vi "F510-X.vi"(7 "Smooth Control (T)":bool=TRUE, 8 "error in (no error)":errorcluster, 10 "Deadzone Scale Cluster":cluster{"Scale":dbl, "Deadzone":dbl}={"Scale"=1.0, "Deadzone"=0.1}, 11 "refnum name":string) -> (0 "error out":errorcluster, 1 "Right Stick":cluster{"X":dbl, "Y":dbl}, 2 "Left Stick":cluster{"X":dbl, "Y":dbl}, 3 "JoystickDevRef":T2, 4 "Buttons":T1, 5 "Triggers":cluster{"Left":dbl, "Right":dbl}, 6 "D-Pad Buttons":T4)   [LabVIEW 2015]
uses:
  <vilib>/Rock Robotics/WPI/Joystick/WPI_JoystickDevRef.ctl
  <vilib>/Rock Robotics/WPI/Joystick/WPI_JoystickDeviceEnum.ctl
  <vilib>/Rock Robotics/WPI/Utilities/WPI_GetSetVariantRefNum.vi
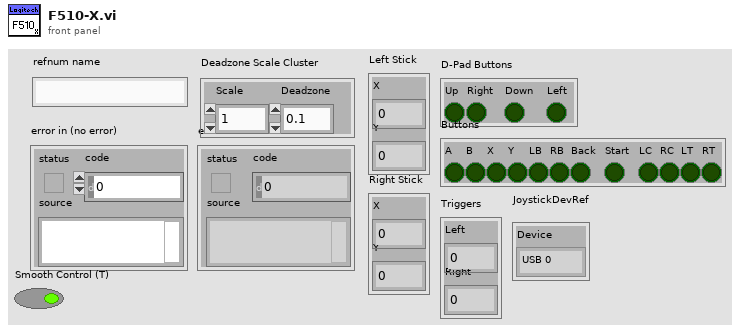
[diagram p1: front panel]
types:
  T1 = cluster{"A":bool, "B":bool, "X":bool, "Y":bool, "LB":bool, "RB":bool, "Back":bool, "Start":bool, "LC":bool, "RC":bool, "LT":bool, "RT":bool}
  T2 = typedef "WPI_JoystickDevRef.ctl" = cluster{"Device":T3}
  T3 = typedef "WPI_JoystickDeviceEnum.ctl" = enum16{"USB 0", "USB 1", "USB 2", "USB 3", "USB 4", "USB 5"}
  T4 = cluster{"Up":bool, "Right":bool, "Down":bool, "Left":bool}
  T5 = cluster{"[0]":dbl, "[1]":dbl, "[2]":dbl, "[3]":dbl, "[4]":dbl, "[5]":dbl}
  T6 = cluster{"Buttons[0]":bool, "Buttons[1]":bool, "Buttons[2]":bool, "Buttons[3]":bool, "Buttons[4]":bool, "Buttons[5]":bool, "Buttons[6]":bool, "Buttons[7]":bool, "Buttons[8]":bool, "Buttons[9]":bool}
  T7 = cluster{"Up":bool, "Down":bool, "Left":bool, "Right":bool}[]
  T8 = cluster{"Up":bool, "Down":bool, "Left":bool, "Right":bool}
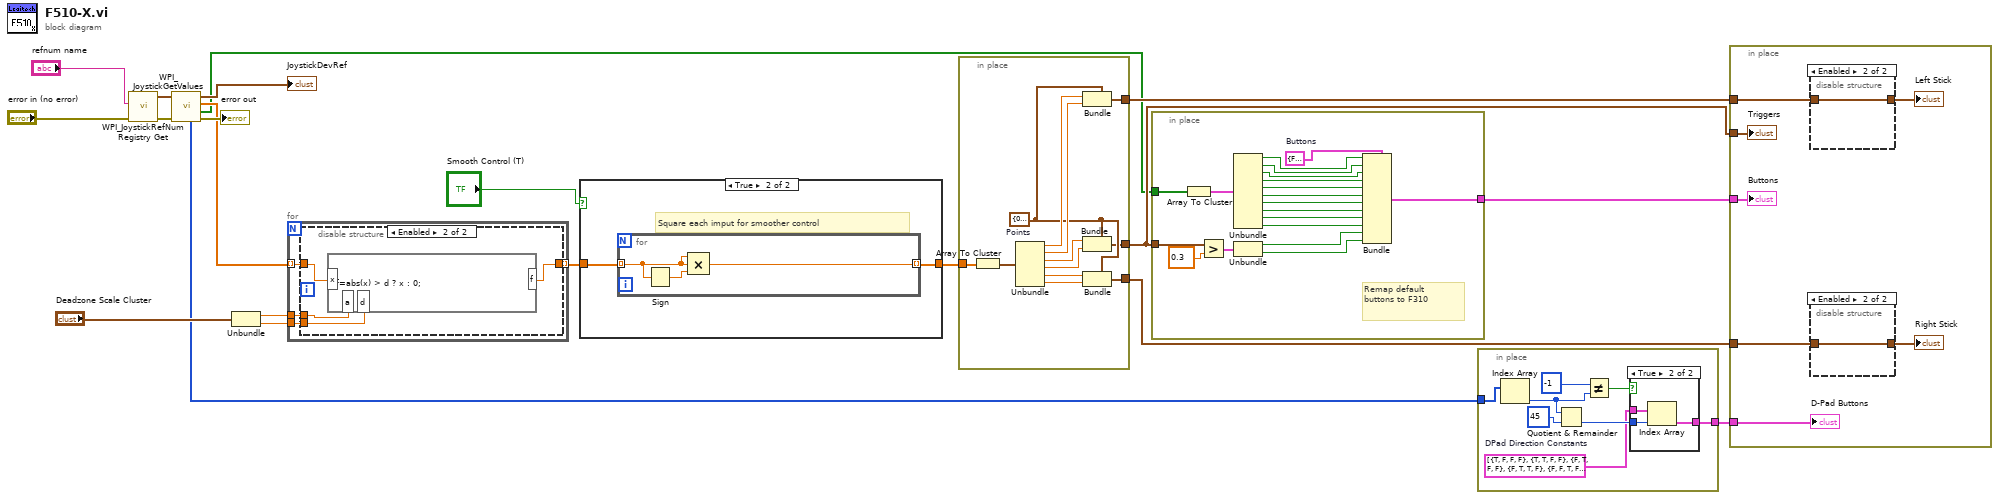
[diagram p0: block diagram]
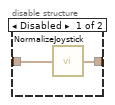
[diagram p3: hidden frame]
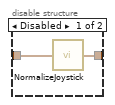
[diagram p4: hidden frame]
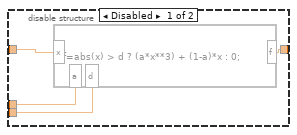
[diagram p6: hidden frame]
diagram:
  n1 = call <vilib>:"WPI_JoystickRefNum Registry Get.vi"("error in (no error)"="error in (no error)", "refnum name"="refnum name") -> ("error out"=w17:errorcluster, "JoystickDevRef"=w18:T2)  [unwired: 8 in]
  n2 = call <vilib>:"WPI_JoystickGetValues.vi"("error in (no error)"=w17, "JoystickDevRef"=w18) -> ("error out"=→"error out":errorcluster, "Buttons"=w5:bool[], "Axes"=w15:dbl[], "JoystickDevRef"=→"JoystickDevRef":T2, "POVs"=w9:i16[])  [unwired: 5 in]
  n3 = Unbundle("Deadzone Scale Cluster") -> ("Scale"=w13:dbl, "Deadzone"=w12:dbl)
  n4 = for {
    tunnel: w15 -> [w24] mode=indexing
    tunnel: w13 -> [w23]
    tunnel: w12 -> [w22]
    tunnel: [w21] -> w1 mode=indexing
    n5 = disable-structure shown="Enabled" {
      disable-tunnel: w24 -> [w28 w30]
      disable-tunnel: w23 -> [w27 w32]
      disable-tunnel: w22 -> [w26 w31]
      disable-tunnel: [w25 w29] -> w21
      frame Disabled {
        n6 = formula code="f=abs(x) > d ? (a*x**3) + (1-a)*x : 0;"("x"=w28, "d"=w26, "a"=w27) -> ("f"=w25:dbl)
      }
      frame Enabled {
        n7 = formula code="f=abs(x) > d ? x : 0;"("x"=w30, "d"=w31, "a"=w32) -> ("f"=w29:dbl)
      }
    }
  }
  n8 = case shown="True" "Smooth Control (T)" {
    tunnel: [w33 w35] -> w2
    tunnel: w1 -> [w33 w34]
    frame False {
    }
    frame True {
      # "Square each imput for smoother control"
      n9 = for {
        tunnel: [w38] -> w35 mode=indexing
        tunnel: w34 -> [w37] mode=indexing
        n10 = Sign(1:w37) -> (0:w36:dbl)
        n11 = Compound Arithmetic op=MULTIPLY(w37, w37, w36) -> (w38:dbl)
      }
    }
  }
  n12 = in-place {
    in-place-border: w2 -> [w47]
    in-place-border: [w43] -> w10
    in-place-border: [w46] -> w11
    in-place-border: [w41] -> w8
    w42 = cluster{"X":dbl, "Y":dbl} {"X"=0.0, "Y"=0.0}  # Points
    n13 = Array To Cluster(array=w47) -> (cluster=w50:T5)
    n14 = Unbundle(w50) -> ("[0]"=w48:dbl, "[1]"=w49:dbl, "[2]"=w40:dbl, "[3]"=w39:dbl, "[4]"=w45:dbl, "[5]"=w44:dbl)
    n15 = Bundle(cluster=w42, "X"=w48, "Y"=w49) -> (w46:cluster{"X":dbl, "Y":dbl})
    n16 = Bundle(cluster=w42, "X"=w40, "Y"=w39) -> (w41:cluster{"X":dbl, "Y":dbl})
    n17 = Bundle(cluster=w42, "X"=w45, "Y"=w44) -> (w43:cluster{"X":dbl, "Y":dbl})
  }
  n18 = in-place {
    in-place-border: w5 -> [w60]
    in-place-border: [w62] -> w4
    in-place-border: w8 -> [w55]
    w69 = T1 {"A"=FALSE, "B"=FALSE, "X"=FALSE, "Y"=FALSE, "LB"=FALSE, "RB"=FALSE, "Back"=FALSE, "Start"=FALSE, "LC"=FALSE, "RC"=FALSE, "LT"=FALSE, "RT"=FALSE}  # Buttons
    # "Remap default\nbuttons to F310"
    n19 = Array To Cluster(array=w60) -> (cluster=w61:T6)
    n20 = Greater?(x=w55, y=0.3) -> (0:w53:cluster{"X":bool, "Y":bool})
    n21 = Unbundle(w61) -> ("Buttons[0]"=w68:bool, "Buttons[1]"=w67:bool, "Buttons[2]"=w66:bool, "Buttons[3]"=w65:bool, "Buttons[4]"=w64:bool, "Buttons[5]"=w63:bool, "Buttons[6]"=w59:bool, "Buttons[7]"=w58:bool, "Buttons[8]"=w57:bool, "Buttons[9]"=w56:bool)
    n22 = Unbundle(w53) -> ("X"=w52:bool, "Y"=w51:bool)
    n23 = Bundle(cluster=w69, "A"=w68, "B"=w67, "X"=w66, "Y"=w65, "LB"=w64, "RB"=w63, "Back"=w59, "Start"=w58, "LC"=w57, "RC"=w56, "LT"=w52, "RT"=w51) -> (w62:T1)
  }
  n24 = in-place {
    in-place-border: w9 -> [w77]
    in-place-border: [w72] -> w7
    w73 = T7 [{"Up"=TRUE, "Down"=FALSE, "Left"=FALSE, "Right"=FALSE}, {"Up"=TRUE, "Down"=TRUE, "Left"=FALSE, "Right"=FALSE}, {"Up"=FALSE, "Down"=TRUE, "Left"=FALSE, "Right"=FALSE}, {"Up"=FALSE, "Down"=TRUE, "Left"=TRUE, "Right"=FALSE}, {"Up"=FALSE, "Down"=FALSE, "Left"=TRUE, "Right"=FALSE}, {"Up"=FALSE, "Down"=FALSE, "Left"=TRUE, "Right"=TRUE}, {"Up"=FALSE, "Down"=FALSE, "Left"=FALSE, "Right"=TRUE}, {"Up"=TRUE, "Down"=FALSE, "Left"=FALSE, "Right"=TRUE}]  # DPad Direction Constants
    n25 = Index Array(array=w77) -> (element=w71:i16)  [unwired: 1 in]
    n26 = Quotient & Remainder(x=w71, y=u16 45) -> (floor(x/y)=w75:u16)  [unwired: 1 out]
    n27 = Not Equal?(x=i16 -1, y=w71) -> (x != y?=w74:bool)
    n28 = case shown="True" w74 {
      tunnel: w75 -> [_ w80]
      tunnel: w73 -> [_ w79]
      tunnel: [_ w78] -> w72
      frame False {
      }
      frame True {
        n29 = Index Array(array=w79, index=w80) -> (element=w78:T8)
      }
    }
  }
  n30 = in-place {
    in-place-border: w11 -> [w84]
    in-place-border: w10 -> [w82]
    in-place-border: w8 -> [w87]
    in-place-border: w7 -> [w86]
    in-place-border: w4 -> [w85]
    n31 = disable-structure shown="Enabled" {
      disable-tunnel: w84 -> [w92 w93]
      disable-tunnel: [w91 w93] -> w83
      frame Disabled {
        n32 = call "NormalizeJoystick.vi"("joystick"=w92) -> ("normalized joystick"=w91:cluster{"x":dbl, "y":dbl})
      }
      frame Enabled {
      }
    }
    "Left Stick" <- w83
    n33 = disable-structure shown="Enabled" {
      disable-tunnel: w82 -> [w89 w90]
      disable-tunnel: [w88 w90] -> w81
      frame Disabled {
        n34 = call "NormalizeJoystick.vi"("joystick"=w89) -> ("normalized joystick"=w88:cluster{"x":dbl, "y":dbl})
      }
      frame Enabled {
      }
    }
    "Right Stick" <- w81
    "Triggers" <- w87
    "D-Pad Buttons" <- w86
    "Buttons" <- w85
  }
